vi "ConvertTimeString.vi"(1 "String":string) -> (0 "time stamp":timestamp)   [LabVIEW 2014]
uses:
  <vilib>/Utility/miscctls.llb/LVDateTimeRec.ctl
panel:
  out "output cluster":T1
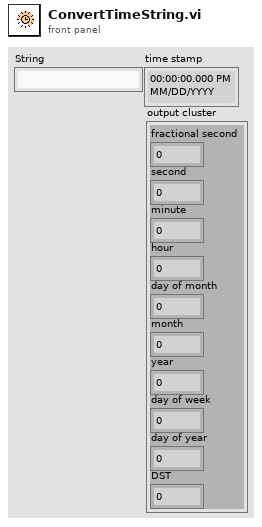
[diagram p1: front panel]
types:
  T1 = typedef "LVDateTimeRec.ctl" = cluster{"fractional second":dbl, "second":i32, "minute":i32, "hour":i32, "day of month":i32, "month":i32, "year":i32, "day of week":i32, "day of year":i32, "DST":i32}
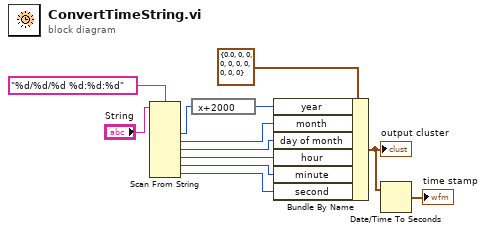
[diagram p0: block diagram]
diagram:
  n1 = Scan From String(format string="%d/%d/%d %d:%d:%d", input string="String") -> (output 1=w9:i32, output 2=w5:i32, output 3=w10:i32, output 4=w11:i32, output 5=w12:i32, output 6=w4:i32)  [unwired: 8 in, 3 out]
  n2 = expression code="x+2000"(w9) -> (w1:i32)
  n3 = Bundle By Name(cluster=T1 {"fractional second"=0.0, "second"=0, "minute"=0, "hour"=0, "day of month"=0, "month"=0, "year"=0, "day of week"=0, "day of year"=0, "DST"=0} ("date time rec"), "year"=w1, "month"=w5, "day of month"=w10, "hour"=w11, "minute"=w12, "second"=w4) -> (w2:T1)
  "output cluster" <- w2
  n4 = Date/Time To Seconds(2:w2) -> (0:→"time stamp":timestamp)  [unwired: 1 in]
